vi "读取探头文件.vi"(11 "字符串":string) -> (3 "all rows":string[][](array[string]) caption="所有行")   [LabVIEW 2021]
uses:
  <vilib>/Utility/file.llb/Read Delimited Spreadsheet (string).vi
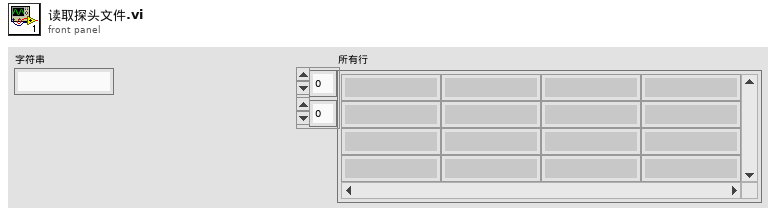
[diagram p1: front panel]
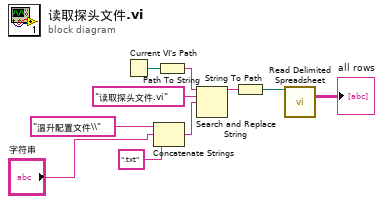
[diagram p0: block diagram]
diagram:
  n1 = Current VI's Path() -> (path=w9:path)
  n2 = Concatenate Strings("温升配置文件\\" ("字符串"), "字符串", ".txt" ("字符串")) -> (w6:string)
  n3 = Path To String(path=w9) -> (string=w8:string)
  n4 = Search and Replace String(input string=w8, search string="读取探头文件.vi" ("搜索字符串"), replace string=w6) -> (result string=w4:string)  [unwired: 5 in, 3 out]
  n5 = String To Path(string=w4) -> (path=w3:path)
  n6 = call-poly <vilib>:"Read Delimited Spreadsheet.vi"("file path (dialog if empty)"=w3) -> ("all rows"=→"all rows":string[][])  [unwired: 9 in, 5 out]
